vi "SysInit.vi"(8 "error in (no error)":errorcluster, 11 "Cluster":T1) -> (0 "error out":errorcluster, 3 "output cluster":T1)   [LabVIEW 2013]
uses:
  Control/SystemProcess.ctl
  Control/SystemTab.ctl
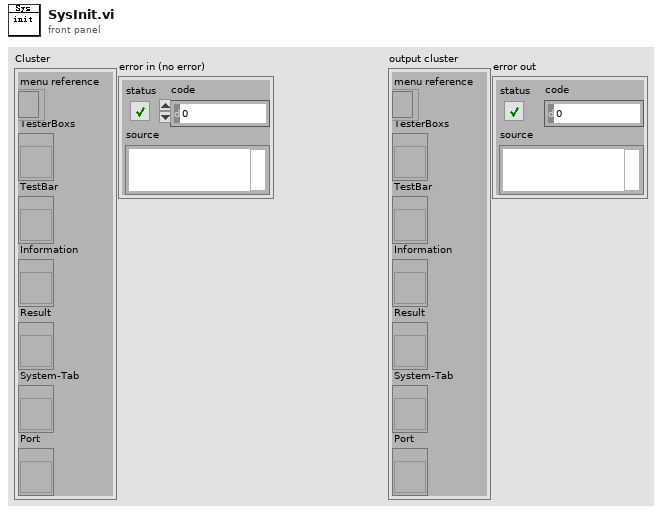
[diagram p1: front panel]
types:
  T1 = cluster{"menu reference":refnum<k9>, "TesterBoxs":refnum<vi>, "TestBar":refnum<vi>, "Information":refnum<vi>, "Result":refnum<vi>, "System-Tab":refnum<vi>, "Port":refnum<vi>}
  T2 = typedef "SystemTab.ctl" = enum32{"Tester", "Set", "Reserve"}
  T3 = typedef "SystemProcess.ctl" = enum16{"Idle", "SystemInit", "SpecialEvent", "Barcode(SN)", "TestInitialize", "Test", "Stop", "SaveTestData", "Exit"}
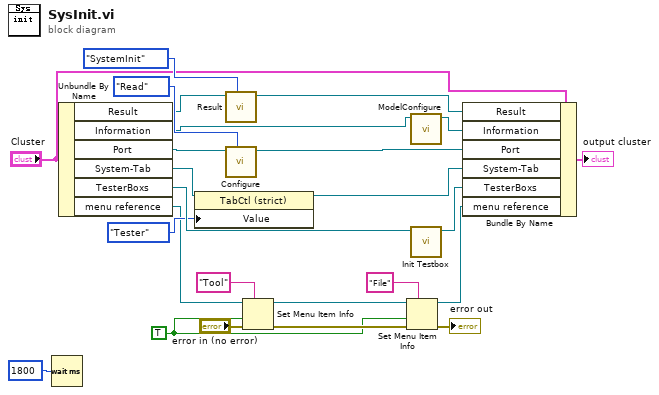
[diagram p0: block diagram]
diagram:
  w7 = TRUE ("enabled")
  n1 = Wait (ms)(milliseconds to wait=u32 1800) -> ()  [unwired: 1 out]
  n2 = Unbundle By Name("Cluster") -> ("Result"=w16:refnum<vi>, "Information"=w14:refnum<vi>, "Port"=w18:refnum<vi>, "System-Tab"=w21:refnum<vi>, "TesterBoxs"=w24:refnum<vi>, "menu reference"=w6:refnum<k9>)
  n3 = property class="TabCtl (strict)"(reference=w21, "Value"=SystemTab."Tester") -> (reference out=w22:refnum<vi>)  [unwired: 1 in, 1 out]
  n4 = call "Result.vi"("MainProcess"=SystemProcess."SystemInit", "Result"=w16) -> ("Result"=w17:refnum<vi>)  [unwired: 9 in]
  n5 = call "Configure.vi"("Enum"=enum16{"Read", "Write"}."Read", "Port 4"=w18) -> ("Port 5"=w19:refnum<vi>)  [unwired: 9 in]
  n6 = Set Menu Item Info(7:"Tool" ("item tag"), 8:"error in (no error)", 9:w7, 11:w6) -> (0:w9:errorcluster, 3:w10:refnum<k9>)  [unwired: 3 in]
  n7 = Set Menu Item Info(7:"File" ("item tag"), 8:w9, 9:w7, 11:w10) -> (0:→"error out":errorcluster, 3:w5:refnum<k9>)  [unwired: 3 in]
  n8 = call "ModelConfigure.vi"("Cluster in"=w14) -> ("Cluster out"=w13:refnum<vi>)  [unwired: 10 in]
  n9 = call "Init Testbox.vi"("MulticolumnListbox in"=w24) -> ("MulticolumnListbox in"=w25:refnum<vi>)  [unwired: 10 in]
  n10 = Bundle By Name(cluster="Cluster", "Result"=w17, "Information"=w13, "Port"=w19, "System-Tab"=w22, "TesterBoxs"=w25, "menu reference"=w5) -> (→"output cluster":T1)
